vi "Shared Get Object Pointer.vi"(11 "Tree in":refnum<class "Tree.lvclass">) -> (1 "Object Pointer":i64, 2 "Assigned object pointer?":bool, 3 "Tree out":refnum<class "Tree.lvclass">)   [LabVIEW 2012, in "MDSplus.lvlib" / "Tree.lvclass"]
uses:
  <vilib>/MDSplus/Classes/Tree_Class/Tree.lvclass
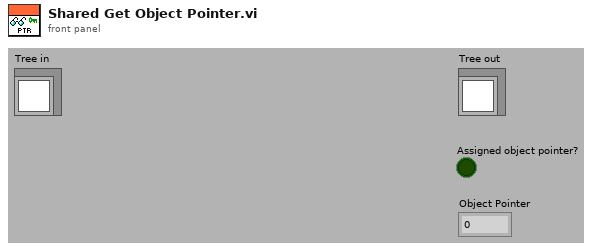
[diagram p1: front panel]
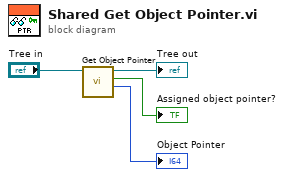
[diagram p0: block diagram]
diagram:
  n1 = call-dynamic "Get Object Pointer.vi"("Tree in"="Tree in") -> ("Object Pointer"=→"Object Pointer":i64, "Assigned object pointer?"=→"Assigned object pointer?":bool, "Tree out"=→"Tree out":refnum<class "Tree.lvclass">)  [unwired: 8 in]
